vi "COMI Error String.vi"(11 "nErrCode":i32) -> (3 "function return":i8)   [LabVIEW 2017, in "Comidll.lvlib"]
doc: "const char (COMI_ErrorString) (int nErrCode);"
uses:
  <userlib>/Comidll/Comidll.lvlib
  <userlib>/Comidll/Comidll.dll
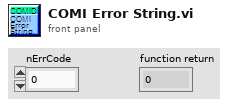
[diagram p1: front panel]
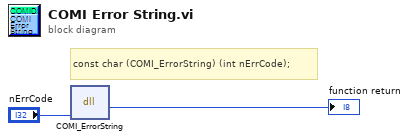
[diagram p0: block diagram]
diagram:
  # "const char (COMI_ErrorString) (int nErrCode);"
  n1 = dll-call lib="C:/Program Files/National Instruments/LabVIEW 2017/user.lib/Comidll/Comidll.*" fn="COMI_ErrorString"("nErrCode"="nErrCode") -> (→"function return":i8)  [unwired: 4 in, 2 out]
